vi "Find All Accessible SLSC Switch CDs.vi"(8 "error in (no error)":errorcluster, 11 "Custom device ref in":T1 format="%.0x") -> (0 "error out":errorcluster, 2 "SLSC Switch CD Paths":string[](array[string]), 3 "Custom device ref out":T1 format="%.0x")   [LabVIEW 2017, in "Routing and Faulting System Explorer.lvlib"]
uses:
  Routing and Faulting System Explorer.lvlib
  <vilib>/NI Veristand/Custom Device API/Custom Device Item Ref.ctl
  Shared/Constants.vi
  <vilib>/NI VeriStand/Custom Device API/Custom Device API.lvlib
  <vilib>/NI Veristand/Custom Device Tools/Custom Device Utility Library/Custom Device Utility Library.lvlib
  Shared/Routing and Faulting Shared.lvlib
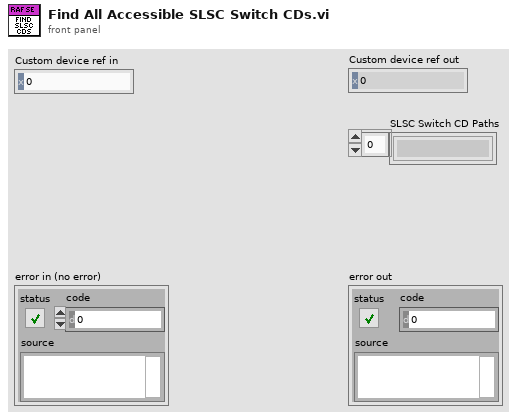
[diagram p1: front panel]
types:
  T1 = typedef "Custom Device API.lvlib/Custom Device Item Ref.ctl" = u64
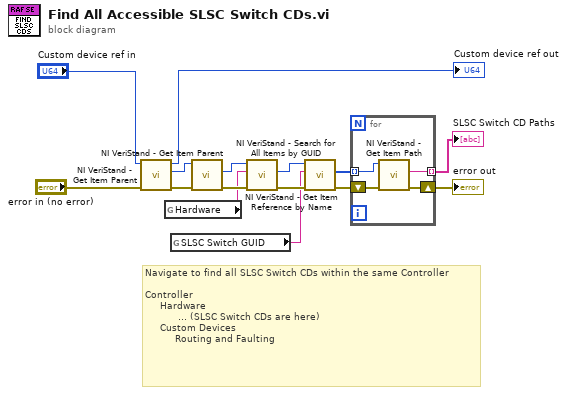
[diagram p0: block diagram]
diagram:
  # "Navigate to find all SLSC Switch CDs within the same Controller\n\nController\n     Hardware\n\t\t         … (SLSC Switch CDs are here)\n     Custom Devices\n          Routing and Faulting"
  n1 = call <vilib>:"NI VeriStand - Get Item Parent.vi"("error in (no error)"="error in (no error)", "Item Ref in"="Custom device ref in") -> ("error out"=w14:errorcluster, "Parent Ref"=w13:T1, "Item Ref out"=→"Custom device ref out":T1)  [unwired: 6 in, 1 out]
  n2 = global read "Constants.vi" "Hardware"() -> (w7:string)
  n3 = global read "Constants.vi" "SLSC Switch GUID"() -> (w8:string)
  n4 = call <vilib>:"NI VeriStand - Get Item Parent.vi"("error in (no error)"=w14, "Item Ref in"=w13) -> ("error out"=w11:errorcluster, "Parent Ref"=w12:T1)  [unwired: 6 in, 2 out]
  n5 = call <vilib>:"NI VeriStand - Get Item Reference by Name.vi"("error in (no error)"=w11, "Item Name"=w7, "Parent Ref in"=w12) -> ("error out"=w9:errorcluster, "Item Ref"=w10:T1)  [unwired: 5 in, 2 out]
  n6 = call <vilib>:"NI VeriStand - Search for All Items by GUID.vi"("error in"=w9, "Item GUID"=w8, "Section Ref in"=w10) -> ("error out"=w5:errorcluster, "Item Refs"=w3:T1[])  [unwired: 5 in, 2 out]
  n7 = for {
    shift-right: [w18] -> w4
    shift-left: w5 -> [w19]
    tunnel: w3 -> [w17] mode=indexing
    tunnel: [w16] -> w2 mode=indexing
    n8 = call <vilib>:"NI VeriStand - Get Item Path.vi"("error in (no error)"=w19, "Item Ref in"=w17) -> ("error out"=w18:errorcluster, "Path"=w16:string)  [unwired: 6 in, 2 out]
  }
  "error out" <- w4
  "SLSC Switch CD Paths" <- w2
